vi "StringToArray.vi"(11 "write buffer":string) -> (3 "Array":string[](array[string]))   [LabVIEW 2017]
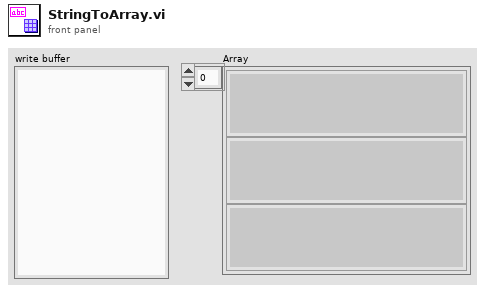
[diagram p1: front panel]
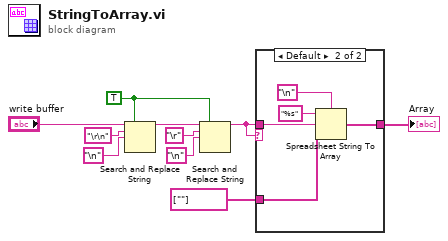
[diagram p0: block diagram]
diagram:
  w3 = TRUE ("replace all? (F)")
  n1 = Search and Replace String(replace all?=w3, input string="write buffer", search string="\r\n", replace string="\n" ("search string")) -> (result string=w4:string)  [unwired: 4 in, 3 out]
  n2 = Search and Replace String(replace all?=w3, input string=w4, search string="\r", replace string="\n" ("search string")) -> (result string=w1:string)  [unwired: 4 in, 3 out]
  n3 = case shown="Default" w1 {
    tunnel: string[] [""] -> [w11 w16]
    tunnel: w1 -> [_ w13]
    tunnel: [w11 w12] -> w2
    frame "" {
    }
    frame Default {
      n4 = Spreadsheet String To Array(delimiter (Tab)="\n", format string="%s", spreadsheet string=w13, array type (2D Dbl)=w16) -> (array=w12:string[])
    }
  }
  "Array" <- w2
